vi "Read Query Value.vi"(8 "error in (no error)":errorcluster, 10 "Query Variable":string, 11 "URI in":refnum<class "URI.lvclass">) -> (0 "error out":errorcluster, 1 "Exists?":bool, 2 "Value":string, 3 "URI out":refnum<class "URI.lvclass">)   [LabVIEW 2020, in "IO.lvlib" / "URI.lvclass"]
uses:
  URI.lvclass
  URI.lvclass/URI.ctl
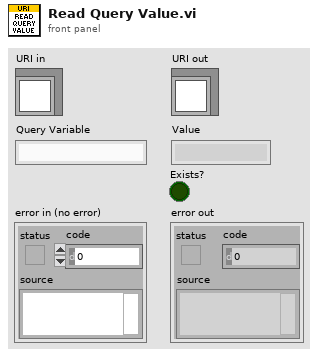
[diagram p1: front panel]
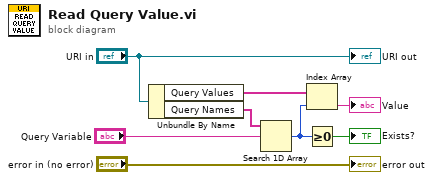
[diagram p0: block diagram]
diagram:
  n1 = Unbundle By Name("URI in") -> ("Query Values"=w4:string[], "Query Names"=w6:string[])
  n2 = Search 1D Array(1D array=w6, element="Query Variable") -> (index of element=w2:i32)  [unwired: 1 in]
  n3 = Index Array(array=w4, index=w2) -> (element=→"Value":string)
  n4 = Greater Or Equal To 0?(x=w2) -> (x >= 0?=→"Exists?":bool)
  "error out" <- "error in (no error)"
  "URI out" <- "URI in"
